vi "example.vi"(8 "error in":errorcluster, 9 "stop":bool, 10 "Multicolumn Listbox":i32(listbox), 11 "Device Name":tag="myDAQ3") -> (3 "Array":dbl[](array[numeric]))   [LabVIEW 2013]
panel:
  out "error out":errorcluster
  out "Value":i32
  out "Measurement":dbl
  out "Waveform Graph":dbl[](graph)
  out "Overrange":u16(ring) items=["In Range", "+Over", "-Over", "±Over"]
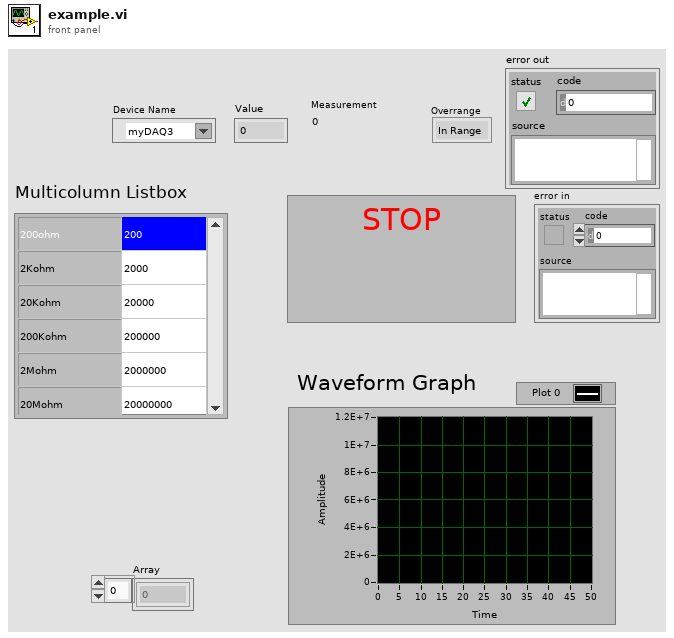
[diagram p1: front panel]
types:
  T1 = typedef "LVRowAndColumnTypeDef.ctl" = cluster{"Row":i32, "Column":i32}
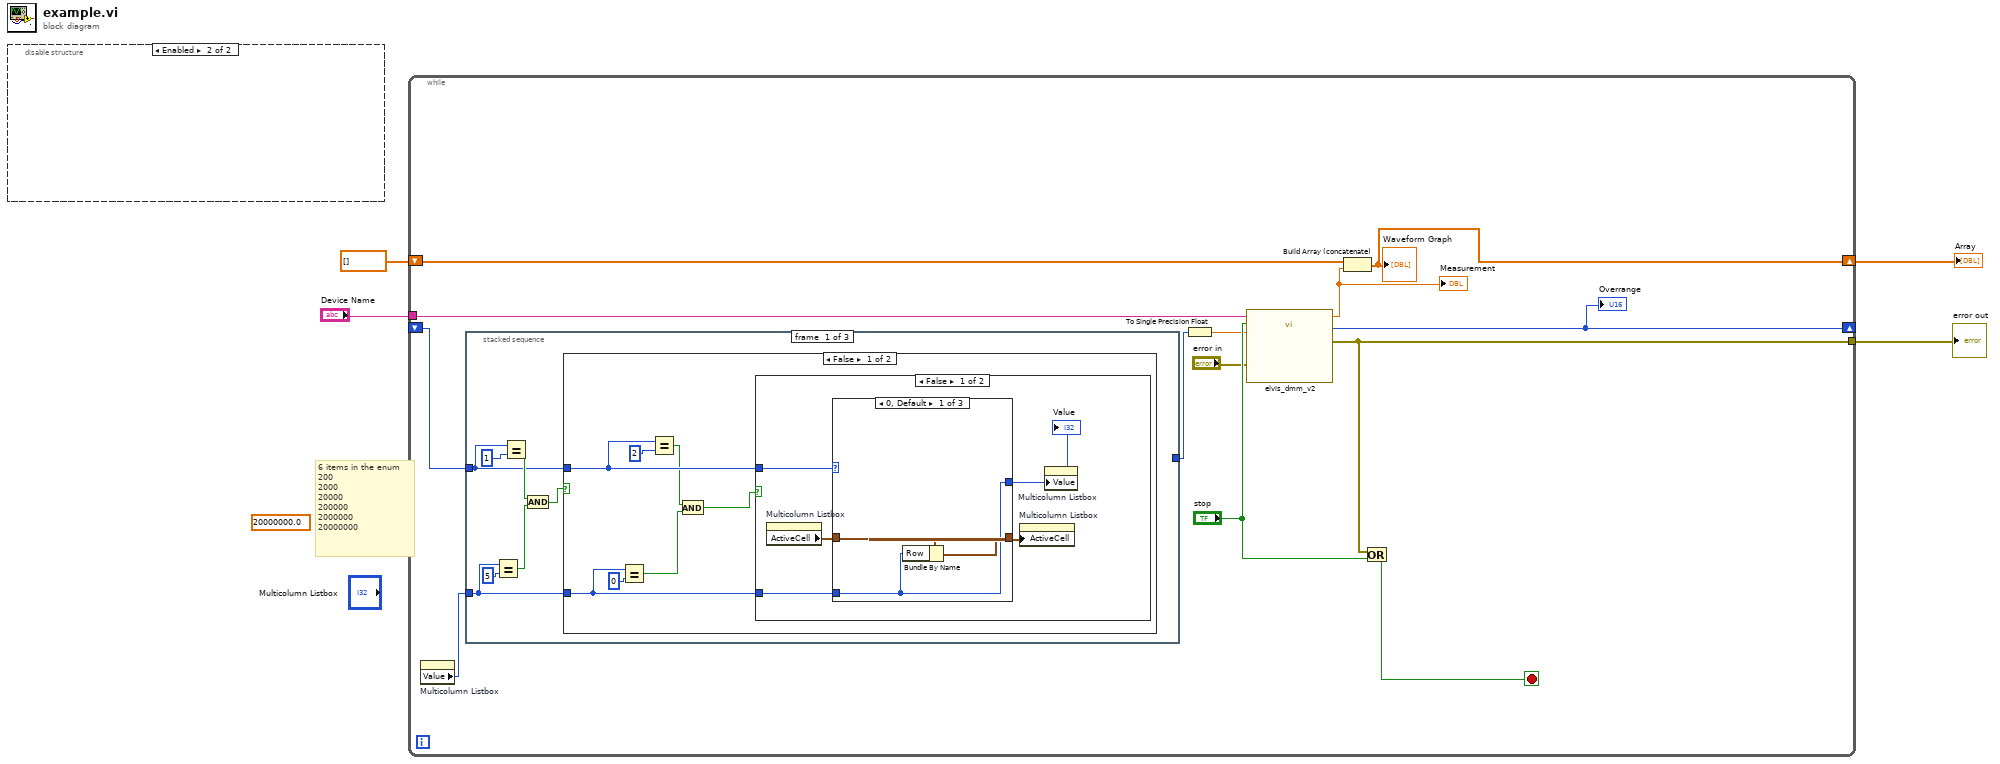
[diagram p0: block diagram]
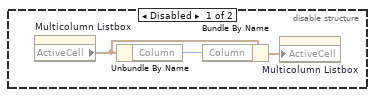
[diagram p2: hidden frame]
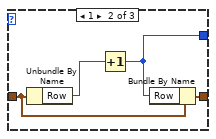
[diagram p3: hidden frame]
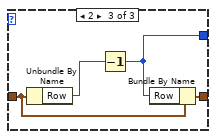
[diagram p4: hidden frame]
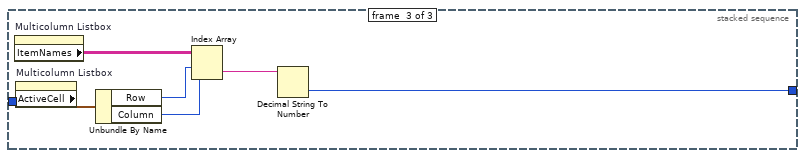
[diagram p8: hidden frame]
diagram:
  (unwired) sgl 20000000.0 items=["200ohm"=200.0, "2Kohm"=2000.0, "20Kohm"=20000.0, "200Kohm"=200000.0, "2Mohm"=2000000.0, "20Mohm"=20000000.0] ("myDAQ Resistance Input Range (Ohms) 2")
  # "6 items in the enum\n200\n2000\n20000\n200000\n2000000\n20000000"
  n1 = disable-structure shown="Enabled" {
    frame Disabled {
      n2 = property on="Multicolumn Listbox" class="MCListbox (strict)"() -> ("ActiveCell"=w6:T1)  [unwired: 2 in, 2 out]
      n3 = Unbundle By Name(w6) -> ("Column"=w7:i32)
      n4 = Bundle By Name(cluster=w6, "Column"=w7) -> (w5:T1)
      n5 = property on="Multicolumn Listbox" class="MCListbox (strict)"("ActiveCell"=w5) -> ()  [unwired: 2 in, 2 out]
    }
    frame Enabled {
    }
  }
  n6 = while {
    tunnel: "Device Name" -> [w20]
    tunnel: [w17] -> w4
    shift-right: [w18] -> w1
    shift-left: dbl[] [] -> [w19]
    shift-right: [w13] -> _
    shift-left: _ -> [w12]
    stop <- w15 stop-if-true
    n7 = property on="Multicolumn Listbox" class="MCListbox (strict)"() -> ("Value"=w9:i32)  [unwired: 2 in, 2 out]
    n8 = stacked-sequence {
      tunnel: w12 -> [w21 _ _]
      tunnel: [_ _ w51] -> w10
      tunnel: w9 -> [w26 _ _]
      frame #0 {
        n9 = Equal?(x=w26, y=5) -> (x = y?=w23:bool)
        n10 = Equal?(x=w21, y=u16 1) -> (x = y?=w24:bool)
        n11 = And(x=w24, y=w23) -> (x .and. y?=w22:bool)
        n12 = case shown="False" w22 {
          tunnel: w26 -> [w32 _]
          tunnel: w21 -> [w33 _]
          frame False {
            n13 = Equal?(x=w32, y=0) -> (x = y?=w29:bool)
            n14 = Equal?(x=w33, y=u16 2) -> (x = y?=w30:bool)
            n15 = And(x=w30, y=w29) -> (x .and. y?=w28:bool)
            n16 = case shown="False" w28 {
              tunnel: w32 -> [w38 _]
              tunnel: w33 -> [w37 _]
              frame False {
                n17 = property on="Multicolumn Listbox" class="MCListbox (strict)"() -> ("ActiveCell"=w39:T1)  [unwired: 2 in, 2 out]
                n18 = case shown="0, Default" w37 {
                  tunnel: w39 -> [w42 w46 w50]
                  tunnel: [w41 w44 w48] -> w36
                  tunnel: w38 -> [w40 _ _]
                  tunnel: [w40 w43 w47] -> w35
                  frame 0, Default {
                    n19 = Bundle By Name(cluster=w42, "Row"=w40) -> (w41:T1)
                  }
                  frame 1 {
                    n20 = Unbundle By Name(w46) -> ("Row"=w45:i32)
                    n21 = Increment(x=w45) -> (x+1=w43:i32)
                    n22 = Bundle By Name(cluster=w46, "Row"=w43) -> (w44:T1)
                  }
                  frame 2 {
                    n23 = Unbundle By Name(w50) -> ("Row"=w49:i32)
                    n24 = Decrement(x=w49) -> (x-1=w47:i32)
                    n25 = Bundle By Name(cluster=w50, "Row"=w47) -> (w48:T1)
                  }
                }
                "Value" <- w35
                n26 = property on="Multicolumn Listbox" class="MCListbox (strict)"("ActiveCell"=w36) -> ()  [unwired: 2 in, 2 out]
                n27 = property on="Multicolumn Listbox" class="MCListbox (strict)"("Value"=w35) -> ()  [unwired: 2 in, 2 out]
              }
              frame True {
              }
            }
          }
          frame True {
          }
        }
      }
      frame #1 {
      }
      frame #2 {
        n28 = property on="Multicolumn Listbox" class="MCListbox (strict)"() -> ("ItemNames"=w56:string[][])  [unwired: 2 in, 2 out]
        n29 = property on="Multicolumn Listbox" class="MCListbox (strict)"() -> ("ActiveCell"=w55:T1)  [unwired: 2 in, 2 out]
        n30 = Unbundle By Name(w55) -> ("Row"=w54:i32, "Column"=w53:i32)
        n31 = Index Array(array=w56, index (row)=w54, index (col)=w53) -> (element=w52:string)
        n32 = Decimal String To Number(string=w52) -> (number=w51:i32)  [unwired: 2 in, 1 out]
      }
    }
    n33 = To Single Precision Float(number=w10) -> (single precision float=w11:sgl)
    n34 = call "elvis_dmm_v2.vi"("Device Name"=w20, "Stop"="stop", "myDAQ Resistance Input Range (Ohms)"=w11, "error in"="error in") -> ("Measurement"=w14:dbl, "Overrange"=w13:u16, "error out"=w17:errorcluster)  [unwired: 13 in]
    "Measurement" <- w14
    "Overrange" <- w13
    n35 = Build Array (concatenate)(w19, w14) -> (w18:dbl[])
    "Waveform Graph" <- w18
    n36 = Or(x=w17, y="stop") -> (x .or. y?=w15:bool)
  }
  "Array" <- w1
  "error out" <- w4
